vi "3_Develope AND NAND OR NOR Gates.vi"() -> ()   [LabVIEW 2018]
panel:
  out "NOR":bool
  out "NAND":bool
  out "AND":bool
  out "OR":bool
  in  "Push Button 2":bool
  in  "Push Button 1":bool
  # "Develope AND NAND OR NOR Gates"
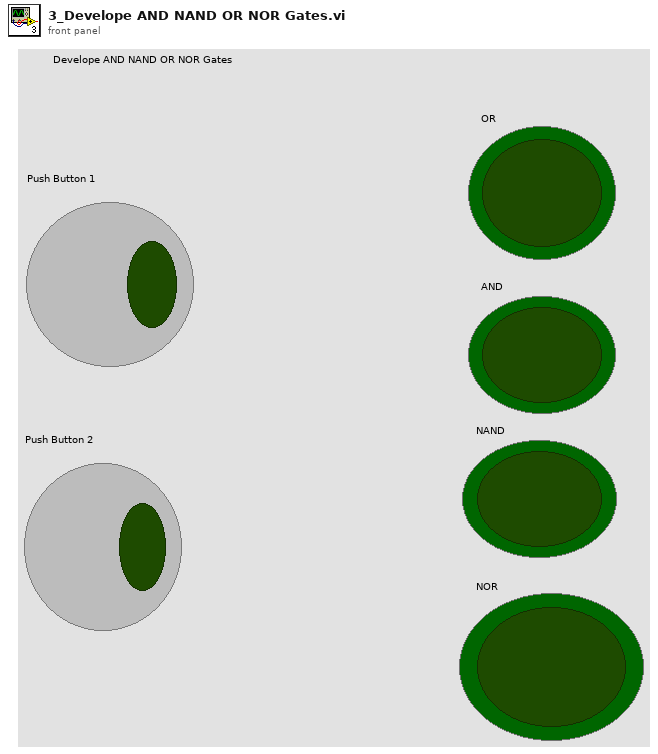
[diagram p1: front panel]
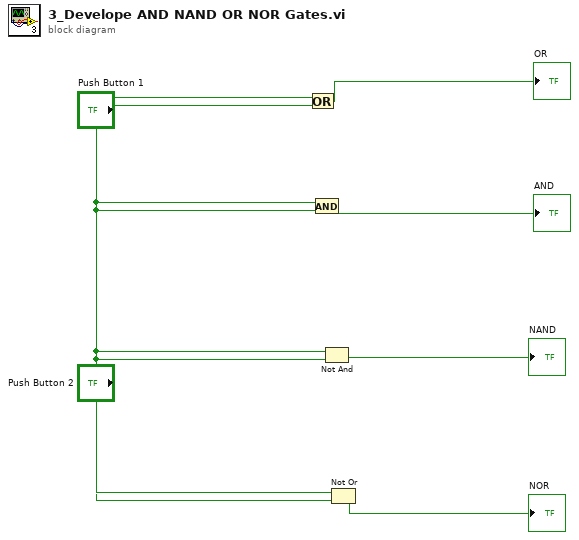
[diagram p0: block diagram]
diagram:
  n1 = Or(x="Push Button 1", y="Push Button 2") -> (x .or. y?=→"OR":bool)
  n2 = And(x="Push Button 1", y="Push Button 2") -> (x .and. y?=→"AND":bool)
  n3 = Not And(1:"Push Button 2", 2:"Push Button 1") -> (0:→"NAND":bool)
  n4 = Not Or(1:"Push Button 2", 2:"Push Button 1") -> (0:→"NOR":bool)
